vi "CE14. Read_Current(subVI).vi"(8 "error in (no error)":errorcluster, 9 "milliseconds to wait(200)":u32=200, 11 "VISA resource name":refnum<visa-resource-name>) -> (0 "error out":errorcluster, 1 "Current (x.xx Amps)":string, 2 "received msg":string, 3 "VISA resource name out":refnum<visa-resource-name>)   [LabVIEW 2018, in "CE14_eMIC.lvlib"]
uses:
  CE14_eMIC.lvlib
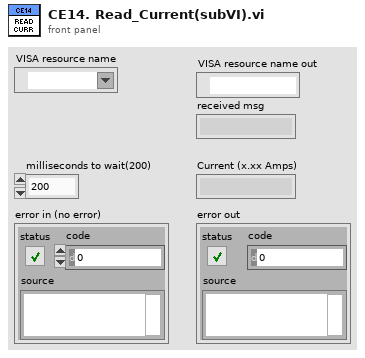
[diagram p1: front panel]
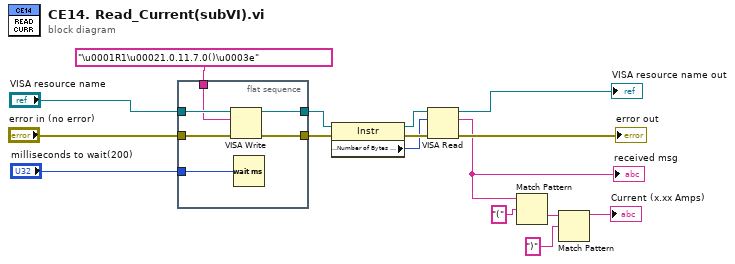
[diagram p0: block diagram]
diagram:
  n1 = flat-sequence {
    tunnel: "VISA resource name" -> [w22]
    tunnel: "error in (no error)" -> [w21]
    tunnel: [w20] -> w13
    tunnel: [w19] -> w11
    tunnel: "milliseconds to wait(200)" -> [w18]
    tunnel: "\u0001R1\u00021.0.11.7.0()\u0003e" -> [w17]
    frame #0 {
      n2 = VISA Write(VISA resource name=w22, write buffer=w17, error in (no error)=w21) -> (VISA resource name out=w19:refnum<visa-resource-name>, error out=w20:errorcluster)  [unwired: 1 out]
      n3 = Wait (ms)(milliseconds to wait=w18) -> ()  [unwired: 1 out]
    }
  }
  n4 = property class="Instr"(reference=w11, error in=w13) -> (reference out=w10:refnum<visa-resource-name>, error out=w12:errorcluster, "Serial Settings:Number of Bytes at Serial Port"=w8:u32)
  n5 = VISA Read(VISA resource name=w10, byte count=w8, error in (no error)=w12) -> (VISA resource name out=→"VISA resource name out":refnum<visa-resource-name>, read buffer=w1:string, error out=→"error out":errorcluster)  [unwired: 1 out]
  "received msg" <- w1
  n6 = Match Pattern(string=w1, regular expression="(") -> (after substring=w3:string)  [unwired: 1 in, 3 out]
  n7 = Match Pattern(string=w3, regular expression=")") -> (before substring=→"Current (x.xx Amps)":string)  [unwired: 1 in, 3 out]
